vi "JTAG SPI Send Data to Stim ASIC.vi"(8 "error in (no error)":errorcluster, 11 "String":string="RECT1\t0x010\t0xFF\nSEQ0A\t0x00C\t0x00\nSEQ0B\t0x00D\t0x00\nPH1.CTL1\t0x040\t0x40\nPH1.CTL2\t0x041\t0x00\nPH1.STPA\t0x042\t0x46\nPH1.STPB\t0x043\t0x03\nPH1.STPC\t0x044\t0x00\nPH1.PG_TIMEOUT\t0x07D\t0x00") -> (0 "error out":errorcluster)   [LabVIEW 2010]
panel:
  out "array":string[][](array[string])
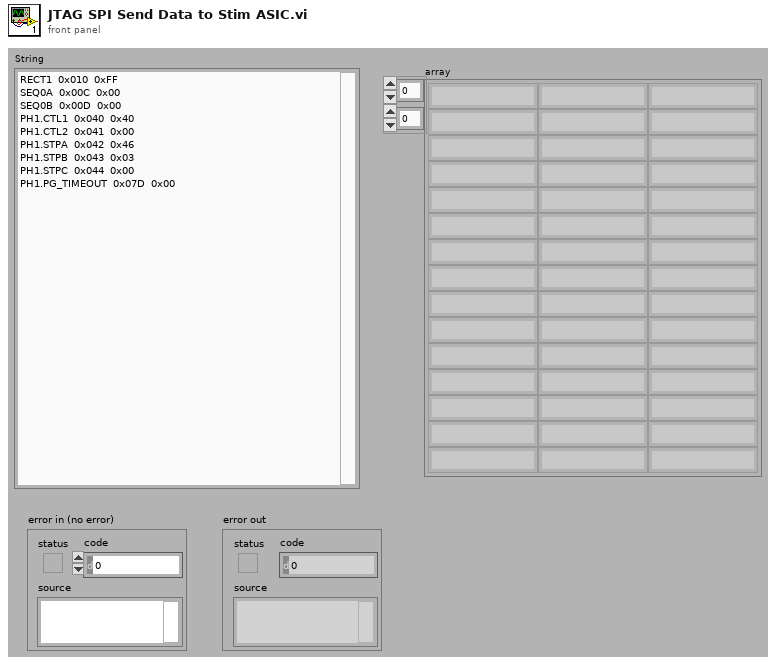
[diagram p1: front panel]
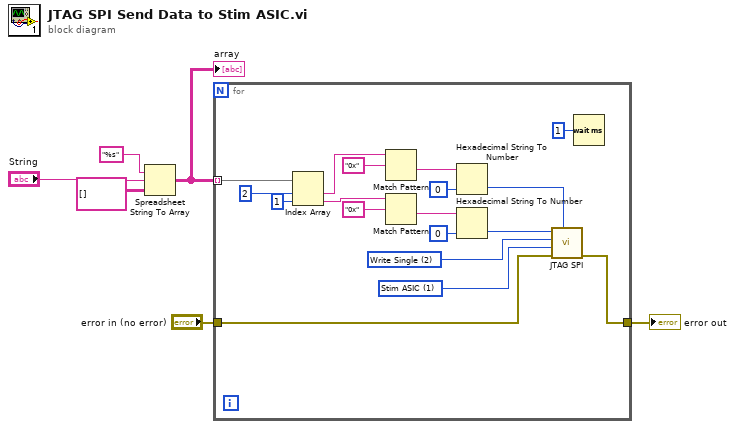
[diagram p0: block diagram]
diagram:
  n1 = Spreadsheet String To Array(format string="%s" ("spreadsheet string"), spreadsheet string="String", array type (2D Dbl)=string[][] []) -> (array=w3:string[][])  [unwired: 1 in]
  "array" <- w3
  n2 = for {
    tunnel: w3 -> [w24] mode=indexing
    tunnel: "error in (no error)" -> [w13]
    tunnel: [w12] -> w1
    w10 = u16 1 items=["Power ASIC", "Stim ASIC", "MICS Radio", "FRAM"] ("Target")
    w11 = u16 2 items=["Power UP", "Power DN", "Write Single", "Read Single", "Write Block", "Read Block", "Write Masked", "Test Value"] ("Function")
    n3 = Index Array(array=w24, index #1=2 ("index"), index #2=1 ("index")) -> (element #1=w16:string, element #2=w18:string)
    n4 = Match Pattern(string=w16, regular expression="0x" ("search string/char (-)")) -> (after substring=w8:string)  [unwired: 1 in, 3 out]
    n5 = Match Pattern(string=w18, regular expression="0x" ("search string/char (-)")) -> (after substring=w9:string)  [unwired: 1 in, 3 out]
    n6 = Hexadecimal String To Number(string=w8, default (0uL)=u8 0 ("default (0 U32)")) -> (number=w14:u8)  [unwired: 1 in, 1 out]
    n7 = Hexadecimal String To Number(string=w9, default (0uL)=u16 0 ("default (0 U32)")) -> (number=w21:u16)  [unwired: 1 in, 1 out]
    n8 = call "JTAG SPI.vi"("Value"=w14, "error in (no error)"=w13, "Target"=w10, "Function"=w11, "Address"=w21) -> ("error out"=w12:errorcluster)  [unwired: 3 in, 3 out]
    n9 = Wait (ms)(milliseconds to wait=u32 1) -> ()  [unwired: 1 out]
  }
  "error out" <- w1
